vi "Launch Programmer.vi"(8 "error in (no error)":errorcluster, 9 "Programming Complete Event":refnum<user-event>, 10 "Position":u32, 11 "Program RF in":refnum<class "Program RF.lvclass">) -> (0 "error out":errorcluster)   [LabVIEW 2015, in "Program RF.lvclass"]
uses:
  Program RF.lvclass
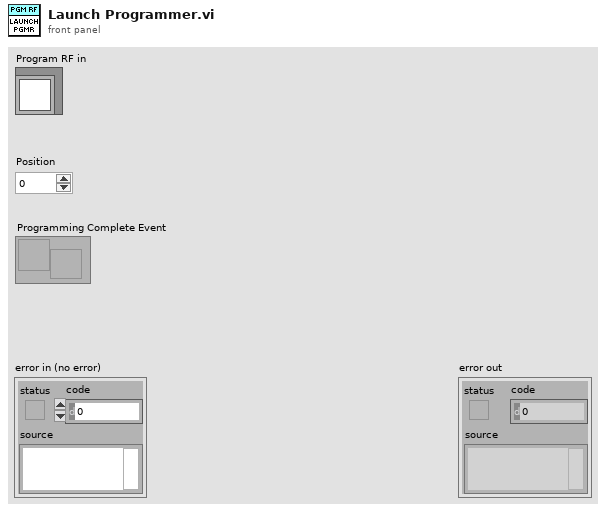
[diagram p1: front panel]
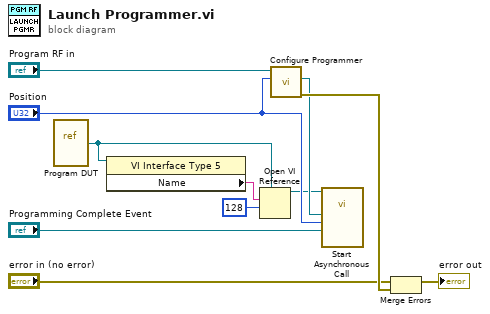
[diagram p0: block diagram]
diagram:
  n1 = vi-ref "Program DUT.vi"() -> (w7:refnum<vi>)
  n2 = property class="VI Interface Type 5"(reference=w7) -> ("Name"=w5:string)  [unwired: 1 in, 2 out]
  n3 = Open VI Reference(type specifier VI Refnum (for type only)=w7, vi path=w5, options=128) -> (vi reference=w4:refnum<vi>)  [unwired: 3 in, 1 out]
  n4 = call-dynamic "Configure Programmer.vi"("Position"="Position", "Program RF in"="Program RF in") -> ("error out"=w11:errorcluster, "Programmer out"=w10:refnum<class "Segger Flasher ARM.lvclass">)  [unwired: 8 in]
  n5 = call-by-ref "Start Asynchronous Call"(reference=w4, "Programming Complete Event"="Programming Complete Event", "Position"="Position", "Programmer"=w10) -> ()  [unwired: 10 in, 2 out]
  n6 = Merge Errors("error in (no error)", w11) -> (→"error out":errorcluster)
